vi "Resample.vi"(7 "Resampling up":bool, 8 "error in":errorcluster, 9 "Slide":refnum<vi>, 10 "New dt":dbl=1.0 format="%#_13g", 11 "Input data":cdb[](array[numeric])) -> (0 "error out":errorcluster, 3 "IQ data":i16[](array[numeric]))   [LabVIEW 2018]
uses:
  <vilib>/measure/maresamp.llb/Resample Waveform (single shot).vi
  <vilib>/measure/maspectr.llb/FFT Spectrum (Mag-Phase) for 1 Chan (CDB).vi
  <vilib>/Analysis/NI_AALPro.lvlib
  <vilib>/measure/NI_MAPro.lvlib
  <vilib>/Analysis/NI_AALBase.lvlib
  <vilib>/Analysis/2dsp.llb/Resample (constant to constant, complex single-channel).vi
panel:
  out "Waveform Graph 4":cluster{"f0":dbl, "df":dbl, "magnitude":dbl[]}[](graph)
  out "Waveform Graph 2":i16[](graph)
  out "Waveform Graph 3":dbl[](graph)
  out "Waveform Graph":sgl[](graph)
  in  "array":csg[](array[numeric])
  out "Constant-to-Constant Resampling (with padding zeros) 3":cluster{"t0":dbl, "dt":dbl, "Y":dbl[]}(graph)
  out "Constant-to-Constant Resampling (with padding zeros) 2":cluster{"t0":dbl, "dt":dbl, "Y":dbl[]}[](graph)
  in  "dt":dbl=2.8 min=0.0
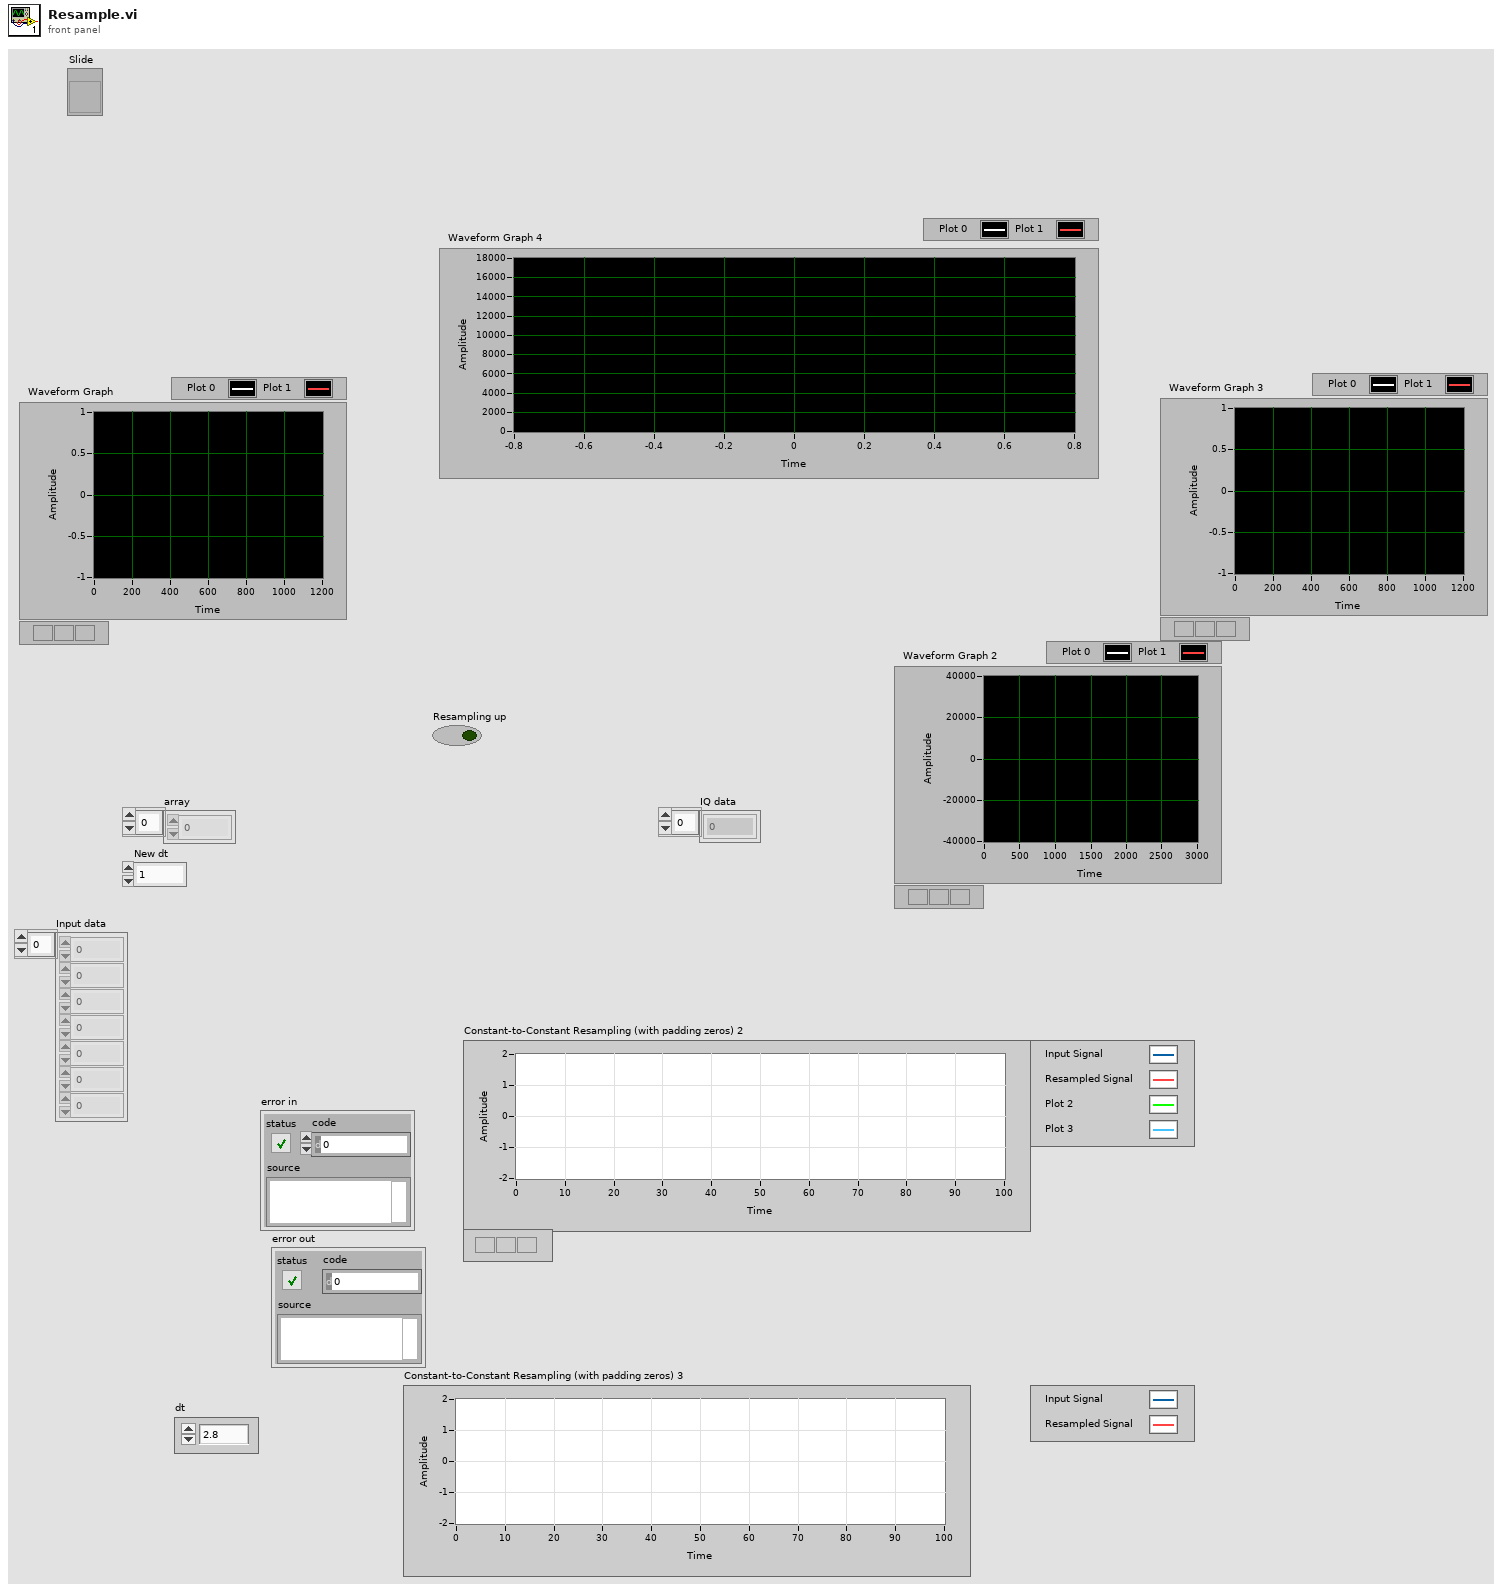
[diagram p1: front panel]
types:
  T1 = cluster{"alias rejection (dB)":dbl, "normalized bandwidth":dbl}
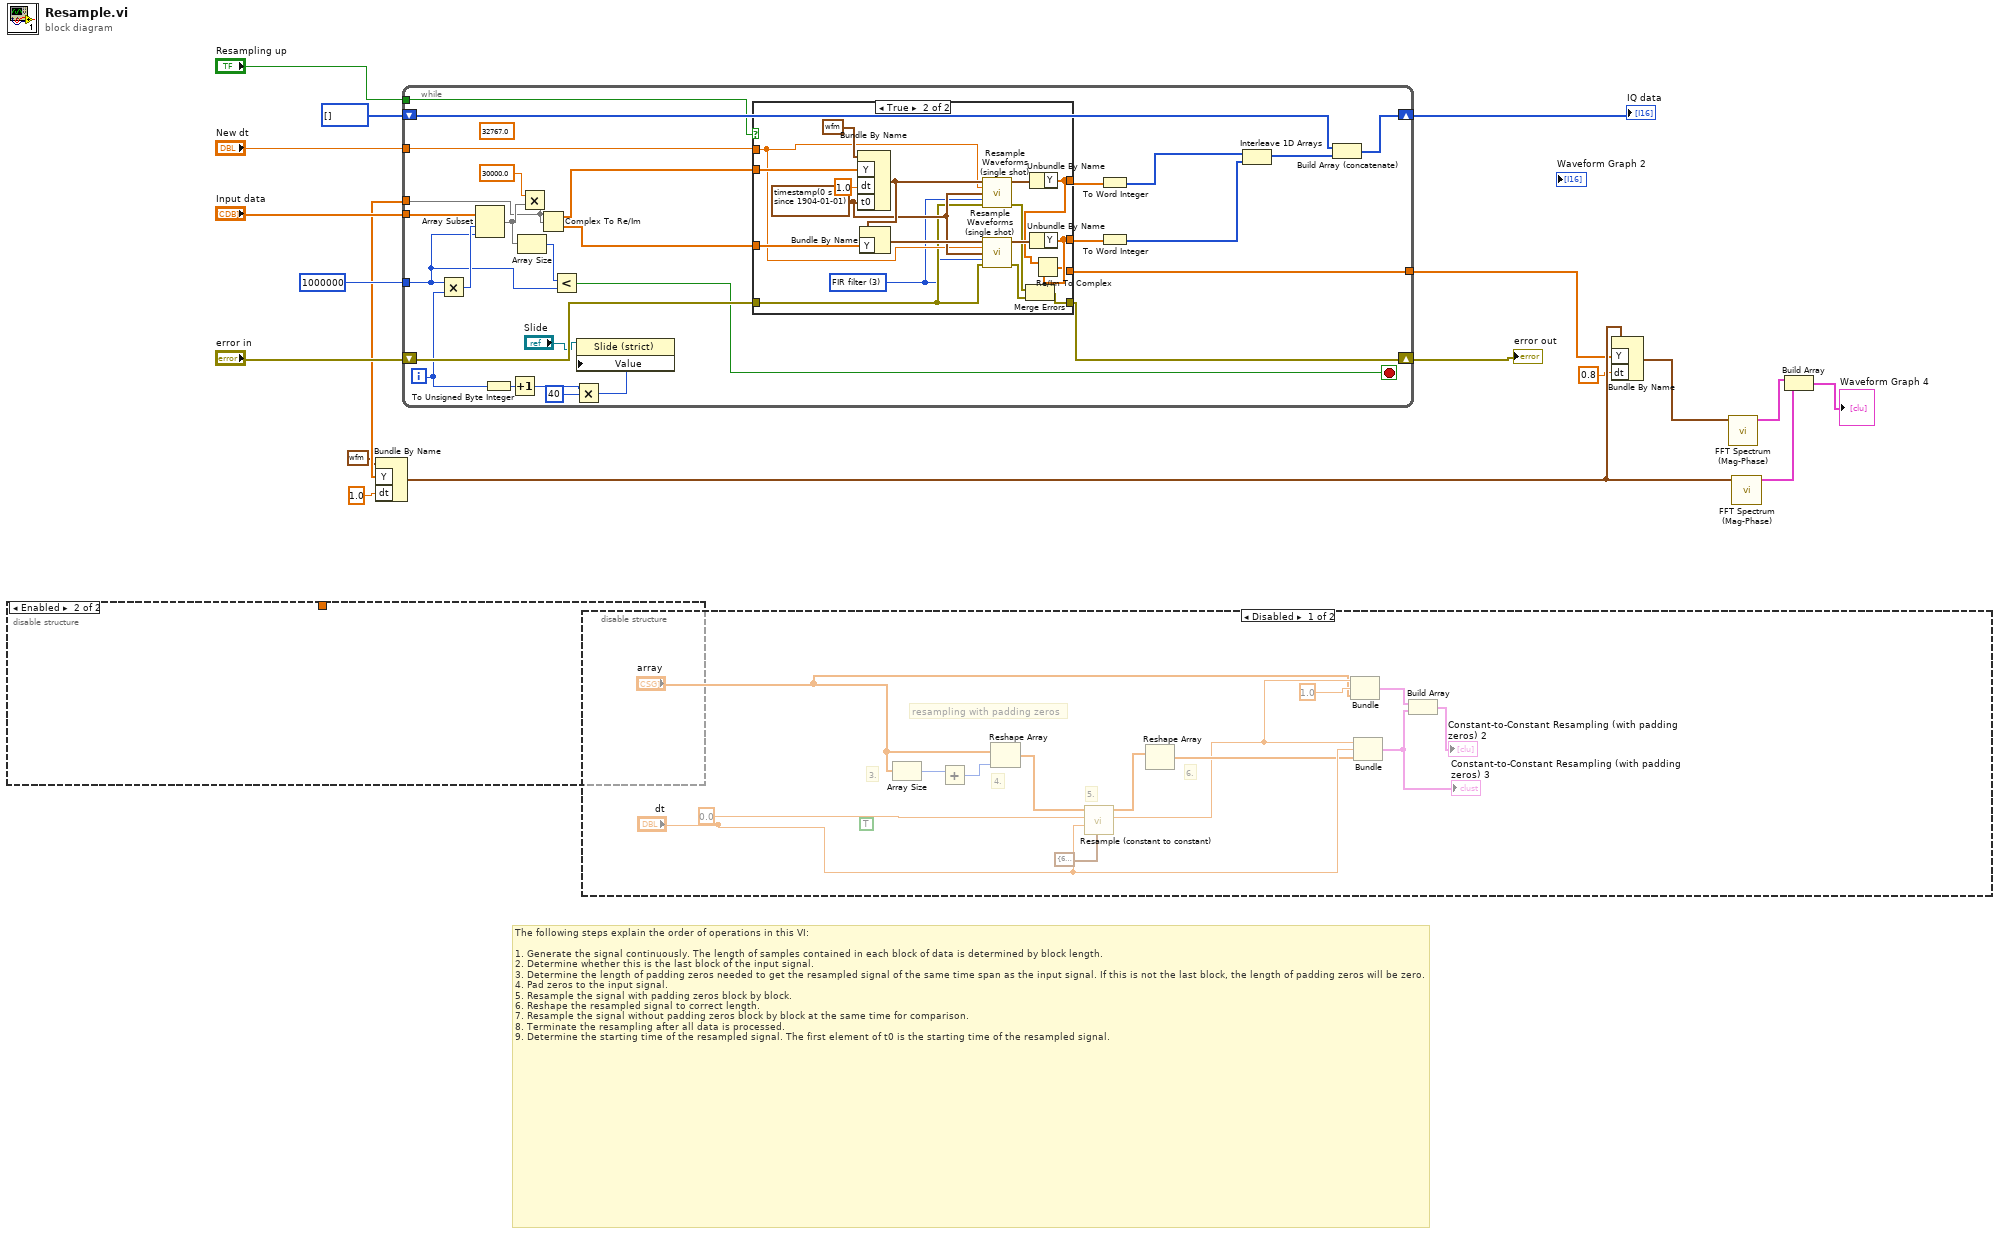
[diagram p0: block diagram]
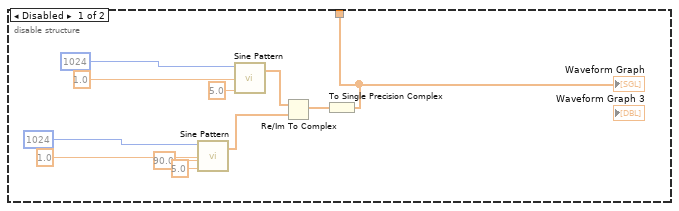
[diagram p2: hidden frame]
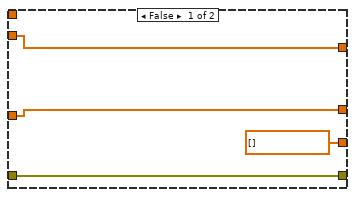
[diagram p3: hidden frame]
diagram:
  # "The following steps explain the order of operations in this VI:\n\n1. Generate the signal continuously. The length of samples contained in each block of data is determined by block length.\n2. Determine whether this is the last block of the input signal.\n3. Determine the length of padding zeros needed to get the resampled signal of the same time span as the input signal. If this is not the last block, the length of padding zeros will be zero. \n4. Pad zeros to the input signal.\n5. Resample the signal with padding zeros block by block.\n6. Reshape the resampled signal to correct length.\n7. Resample the signal without padding zeros block by block at the same time for comparison.\n8. Terminate the resampling after all data is processed.\n9. Determine the starting time of the resampled signal. The first element of t0 is the starting time of the resampled signal."
  n1 = disable-structure shown="Enabled" {
    disable-tunnel: [w19 _] -> _
    frame Disabled {
      n2 = call <vilib>:"Sine Pattern.vi"("cycles"=5.0, "phase(degrees)"=90.0, "amplitude"=1.0, "samples"=1024) -> ("Sinusoidal Pattern"=w21:dbl[])  [unwired: 1 out]
      n3 = call <vilib>:"Sine Pattern.vi"("cycles"=5.0, "amplitude"=1.0, "samples"=1024) -> ("Sinusoidal Pattern"=w22:dbl[])  [unwired: 1 in, 1 out]
      n4 = Re/Im To Complex(1:w21, 2:w22) -> (0:w23:cdb[])
      n5 = To Single Precision Complex(1:w23) -> (0:w19:csg[])
      "Waveform Graph" <- w19
    }
    frame Enabled {
    }
  }
  n6 = while {
    tunnel: 1000000 -> [w54]
    tunnel: "Input data" -> [w57]
    tunnel: "New dt" -> [w51]
    shift-right: [w46] -> w15
    shift-left: "error in" -> [w47]
    shift-right: [w50] -> w1
    shift-left: i16[] [] -> [w49]
    tunnel: "Resampling up" -> [w48]
    tunnel: [w41] -> w11
    tunnel: [w40] -> w7
    i -> [w34]
    stop <- w39 stop-if-true
    (unwired) 32767.0
    n7 = Multiply(x=w54, y=w34) -> (x*y=w56:i32)
    n8 = Array Subset(array=w57, index=w56, length=w54) -> (w44:cdb[])
    n9 = To Unsigned Byte Integer(number=w34) -> (unsigned 8bit integer=w33:u8)
    n10 = Increment(x=w33) -> (x+1=w31:u8)
    n11 = Array Size(array=w44) -> (size(s)=w55:i32)
    n12 = Multiply(x=30000.0, y=w44) -> (x*y=w41:cdb[])
    n13 = Complex To Re/Im(x + iy=w41) -> (x=w53:dbl[], y=w52:dbl[])
    n14 = Less?(x=w55, y=w54) -> (x < y?=w39:bool)
    n15 = Multiply(x=w31, y=u8 40) -> (x*y=w30:u8)
    n16 = property class="Slide (strict)"(reference="Slide", "Value"=w30) -> ()  [unwired: 1 in, 2 out]
    n17 = case shown="True" w48 {
      tunnel: w53 -> [w61 w78]
      tunnel: w52 -> [w60 w77]
      tunnel: w51 -> [_ w72]
      tunnel: w47 -> [w59 w71]
      tunnel: [w61 w64] -> w43
      tunnel: [w60 w63] -> w42
      tunnel: [w59 w66] -> w46
      tunnel: [cdb[] [] w62] -> w40
      frame False {
      }
      frame True {
        w65 = u16 3 items=["coerce", "linear", "spline", "FIR filter"] ("interpolation mode")
        w73 = timestamp(0 s since 1904-01-01) ("t0")
        n18 = Bundle By Name(cluster=waveform(dbl) {"t0"=timestamp(0 s since 1904-01-01), "dt"=1.0, "Y"=[]} ("waveform"), "Y"=w78, "dt"=1.0, "t0"=w73) -> (w76:waveform(dbl))
        n19 = Bundle By Name(cluster=w76, "Y"=w77) -> (w75:waveform(dbl))
        n20 = call-poly <vilib>:"Resample Waveforms (single shot).vi"("waveform in"=w76, "dt"=w72, "t0"=w73, "interpolation mode"=w65, "error in (no error)"=w71) -> ("resampled waveform out"=w70:waveform(dbl), "error out"=w68:errorcluster)  [unwired: 7 in, 2 out]
        n21 = call-poly <vilib>:"Resample Waveforms (single shot).vi"("waveform in"=w75, "dt"=w72, "t0"=w73, "interpolation mode"=w65, "error in (no error)"=w71) -> ("resampled waveform out"=w69:waveform(dbl), "error out"=w67:errorcluster)  [unwired: 7 in, 2 out]
        n22 = Merge Errors(w68, w67) -> (w66:errorcluster)
        n23 = Unbundle By Name(w70) -> ("Y"=w64:dbl[])
        n24 = Unbundle By Name(w69) -> ("Y"=w63:dbl[])
        n25 = Re/Im To Complex(1:w63, 2:w64) -> (0:w62:cdb[])
      }
    }
    n26 = To Word Integer(number=w43) -> (16bit integer=w38:i16[])
    n27 = To Word Integer(number=w42) -> (16bit integer=w36:i16[])
    n28 = Interleave 1D Arrays(w38, w36) -> (w37:i16[])
    n29 = Build Array (concatenate)(w49, w37) -> (w50:i16[])
  }
  "error out" <- w15
  "IQ data" <- w1
  n30 = Bundle By Name(cluster=waveform(cdb) {"t0"=timestamp(0 s since 1904-01-01), "dt"=1.0, "Y"=[]} ("waveform"), "Y"=w11, "dt"=1.0) -> (w8:waveform(cdb))
  n31 = disable-structure shown="Disabled" {
    frame Disabled {
      (unwired) TRUE ("padding zeroes?")
      # "resampling with padding zeros"
      # "6."
      # "5."
      # "4."
      # "3."
      n32 = Array Size(array="array") -> (size(s)=w91:i32)
      n33 = Add(x=w91) -> (x+y=w90:i32)  [unwired: 1 in]
      n34 = Reshape Array("array", w90) -> (w92:csg[])
      n35 = call-poly <vilib>:"Resample (constant to constant).vi"("FIR filter specifications"=T1 {"alias rejection (dB)"=60.0, "normalized bandwidth"=0.4536}, "dt"="dt", "delay"=0.0, "X"=w92) -> ("t0"=w85:dbl, "Y"=w89:cdb[])  [unwired: 5 in, 1 out]
      n36 = Reshape Array(w89) -> (w86:cdb[], w88:i32)
      n37 = Bundle("t0"=w85, "delay"=1.0, "array"="array") -> (w83:cluster{"t0":dbl, "delay":dbl, "array":csg[]})  [unwired: 1 in]
      n38 = Bundle("t0"=w85, "dt"="dt", "Y"=w86) -> (w81:cluster{"t0":dbl, "dt":dbl, "Y":cdb[]})  [unwired: 1 in]
      "Constant-to-Constant Resampling (with padding zeros) 3" <- w81
      n39 = Build Array(w83, w81) -> (→"Constant-to-Constant Resampling (with padding zeros) 2":cluster{"t0":dbl, "dt":dbl, "Y":cdb[]}[])
    }
    frame Enabled {
    }
  }
  n40 = Bundle By Name(cluster=w8, "Y"=w7, "dt"=0.8) -> (w6:waveform(cdb))
  n41 = call-poly <vilib>:"FFT Spectrum (Mag-Phase).vi"("time signal"=w6) -> ("magnitude"=w3:cluster{"f0":dbl, "df":dbl, "magnitude":dbl[]})  [unwired: 6 in, 4 out]
  n42 = call-poly <vilib>:"FFT Spectrum (Mag-Phase).vi"("time signal"=w8) -> ("magnitude"=w2:cluster{"f0":dbl, "df":dbl, "magnitude":dbl[]})  [unwired: 6 in, 4 out]
  n43 = Build Array(w3, w2) -> (→"Waveform Graph 4":cluster{"f0":dbl, "df":dbl, "magnitude":dbl[]}[])
